vi "OpenDBL.vi"(2 "Action":u16(ring) items=["Get Image", "Load and Read File"]) -> (4 "Image":sgl[](array[numeric]), 8 "Physical Length (Z, Y, X, t)":sgl[](array[numeric]), 13 "File Notes":string, 15 "Dimensions (Z, Y, X, t)":i32[](array[numeric]))   [LabVIEW 2014]
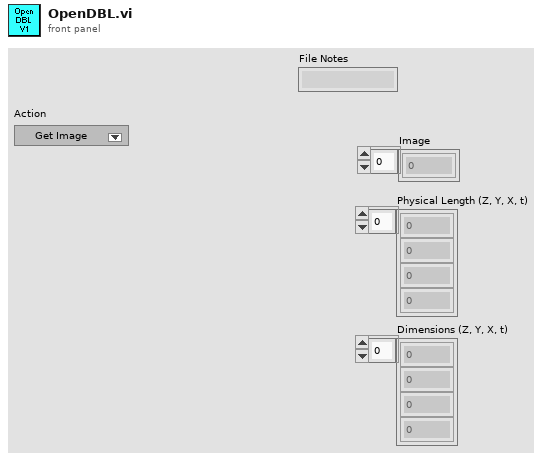
[diagram p1: front panel]
types:
  T1 = enum16{"open", "replace", "create", "open or create", "replace or create", "replace or create with confirmation"}
  T2 = enum16{"big-endian, network order", "native, host order", "little-endian"}
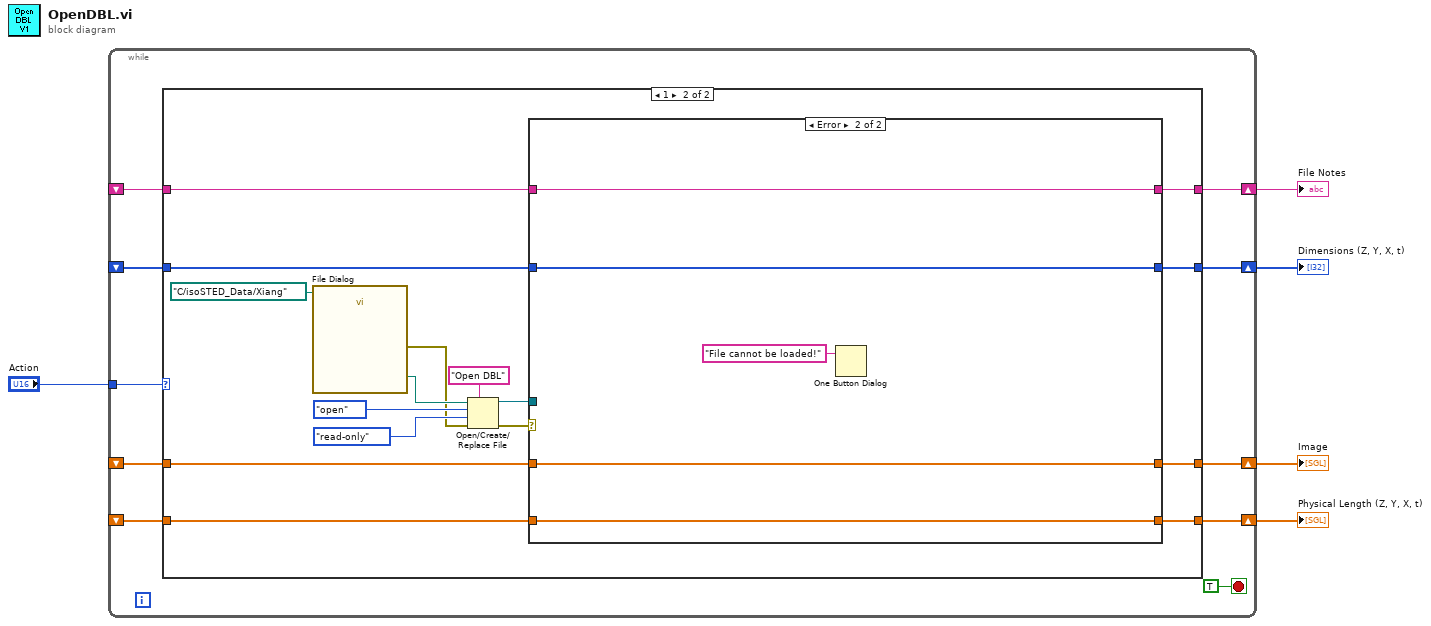
[diagram p0: block diagram]
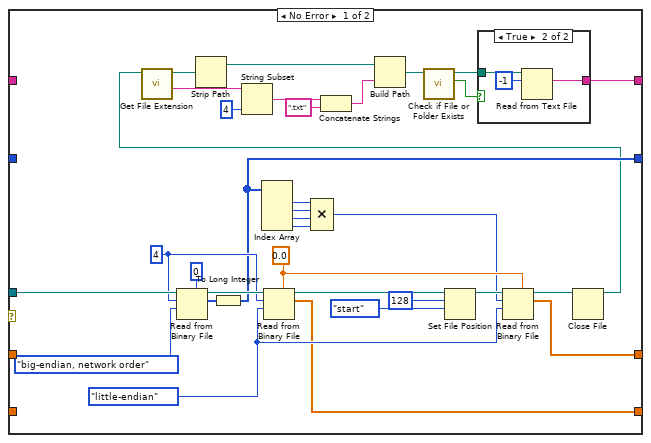
[diagram p3: hidden frame]
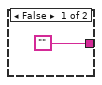
[diagram p4: hidden frame]
diagram:
  n1 = while {
    shift-right: [w13] -> w2
    shift-left: _ -> [w10]
    shift-right: [w11] -> w3
    shift-left: _ -> [w9]
    shift-right: [w12] -> w4
    shift-left: _ -> [w8]
    tunnel: "Action" -> [w14]
    shift-right: [w7] -> w1
    shift-left: _ -> [w6]
    stop <- TRUE stop-if-true
    n2 = case shown="1" w14 {
      tunnel: [w17 w31] -> w12
      tunnel: [w19 w29] -> w13
      tunnel: [w18 w30] -> w11
      tunnel: w10 -> [w19 w22]
      tunnel: w9 -> [w18 w21]
      tunnel: w8 -> [w17 w20]
      tunnel: [w16 w28] -> w7
      tunnel: w6 -> [w16 w23]
      frame 0, Default {
      }
      frame 1 {
        n3 = call "File Dialog"("start path"=path "C:/isoSTED_Data/Xiang") -> ("selected path"=w27:path, "error out"=w25:errorcluster)  [unwired: 11 in, 2 out]
        n4 = Open/Create/Replace File(file path (use dialog)=w27, error in=w25, prompt="Open DBL", operation (0:open)=T1."open", access (0:read/write)=enum16{"read/write", "read-only", "write-only"}."read-only") -> (refnum out=w32:refnum<file>, error out=w24:errorcluster)  [unwired: 1 in, 1 out]
        n5 = case shown="Error" w24 {
          tunnel: w32 -> [w68 _]
          tunnel: [w55 w74] -> w31
          tunnel: [w53 w75] -> w30
          tunnel: [w49 w76] -> w29
          tunnel: [w36 w77] -> w28
          tunnel: w23 -> [_ w77]
          tunnel: w22 -> [_ w76]
          tunnel: w21 -> [_ w75]
          tunnel: w20 -> [_ w74]
          frame No Error {
            w61 = sgl 0.0
            w59 = T2."little-endian" ("byte order (0:big-endian, network order)")
            w62 = 4 ("count (1)")
            n6 = Read from Binary File(5:u16 0, 9:T2."big-endian, network order" ("byte order (0:big-endian, network order)"), 10:w62, 11:w68) -> (2:w54:u16[], 3:w65:refnum<file>)  [unwired: 2 in, 2 out]
            n7 = To Long Integer(number=w54) -> (32bit integer=w49:i32[])
            n8 = Index Array(array=w49) -> (element #1=w50:i32, element #2=w51:i32, element #3=w57:i32, element #4=w56:i32)  [unwired: 4 in]
            n9 = Read from Binary File(5:w61, 9:w59, 10:w62, 11:w65) -> (2:w55:sgl[], 3:w64:refnum<file>)  [unwired: 2 in, 2 out]
            n10 = Compound Arithmetic op=MULTIPLY(w50, w51, w57, w56) -> (w48:i32)
            n11 = Set File Position(offset (in bytes) (0)=i64 128, refnum=w64, from (0:start)=enum16{"start", "end", "current"}."start") -> (refnum out=w52:refnum<file>)  [unwired: 1 in, 1 out]
            n12 = Read from Binary File(5:w61, 9:w59, 10:w48, 11:w52) -> (2:w53:sgl[], 3:w58:refnum<file>)  [unwired: 2 in, 2 out]
            n13 = Close File(refnum=w58) -> (path=w37:path)  [unwired: 1 in, 1 out]
            n14 = call <vilib>:"Get File Extension.vi"("file"=w37) -> ("filename without extension"=w39:string, "dup file"=w38:path)  [unwired: 7 in, 2 out]
            n15 = Strip Path(path=w38) -> (stripped path=w42:path)  [unwired: 1 out]
            n16 = String Subset(string=w39, length (rest)=4 ("length (rest)")) -> (substring=w40:string)  [unwired: 1 in]
            n17 = Concatenate Strings(w40, ".txt" ("string")) -> (w43:string)
            n18 = Build Path(base path=w42, name or relative path=w43) -> (appended path=w45:path)
            n19 = call <vilib>:"Check if File or Folder Exists.vi"("path"=w45) -> ("file or folder exists?"=w47:bool, "dup path"=w46:path)  [unwired: 8 in, 1 out]
            n20 = case shown="True" w47 {
              tunnel: w46 -> [_ w71]
              tunnel: ["" w70] -> w36
              frame False {
              }
              frame True {
                n21 = Read from Text File(file (use dialog)=w71, count=-1) -> (text=w70:string)  [unwired: 2 in, 3 out]
              }
            }
          }
          frame Error {
            n22 = One Button Dialog(message="File cannot be loaded!") -> ()  [unwired: 1 in, 1 out]
          }
        }
      }
    }
  }
  "Dimensions (Z, Y, X, t)" <- w2
  "Physical Length (Z, Y, X, t)" <- w4
  "Image" <- w3
  "File Notes" <- w1
